vi "CoboltLaser_ComPortRead.vi"(0 "ComPort":refnum<visa-resource-name>, 5 "error in (no error)":errorcluster) -> (14 "ComPort Out":refnum<visa-resource-name>, 15 "Response":string, 19 "error out":errorcluster)   [LabVIEW 2012, in "Cobolt.lvclass"]
doc: "Use this template to build a VI to use as a subVI."
uses:
  Template/Cobolt.lvclass
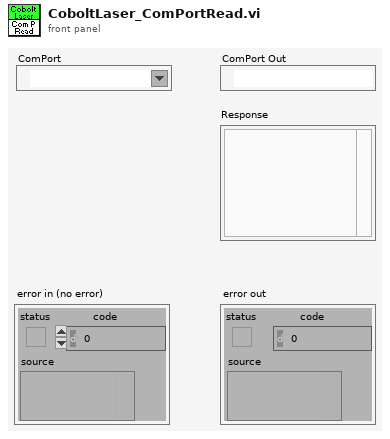
[diagram p1: front panel]
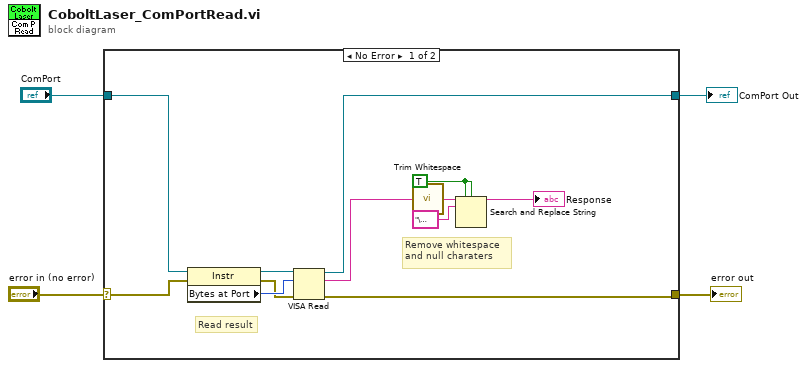
[diagram p0: block diagram]
diagram:
  n1 = case shown="No Error" "error in (no error)" {
    selector: "error in (no error)" -> [w12 w18]
    tunnel: [w13 w18] -> w3
    tunnel: "ComPort" -> [w6 w17]
    tunnel: [w5 w17] -> w1
    frame No Error {
      w9 = TRUE ("replace all? (F)")
      # "Remove whitespace\nand null charaters"
      # "Read result"
      n2 = property class="Instr"(reference=w6, error in=w12) -> (reference out=w16:refnum<visa-resource-name>, error out=w14:errorcluster, "Bytes at Port"=w15:u32)
      n3 = VISA Read(VISA resource name=w16, byte count=w15, error in (no error)=w14) -> (VISA resource name out=w5:refnum<visa-resource-name>, read buffer=w8:string, error out=w13:errorcluster)  [unwired: 1 out]
      n4 = call <vilib>:"Trim Whitespace.vi"("string"=w8) -> ("trimmed string"=w11:string)  [unwired: 1 in]
      n5 = Search and Replace String(replace all?=w9, case sensitive?=w9, input string=w11, search string="\u0000") -> (result string=→"Response":string)  [unwired: 4 in, 3 out]
    }
    frame Error {
    }
  }
  "error out" <- w3
  "ComPort Out" <- w1
